vi "SelectRowTablePaste.vi"(7 "エラー入力":errorcluster, 8 "貼り付け指定行":i32, 9 "部分配列":string[][](array[string]), 10 "Tbl refnum":refnum<vi>) -> (0 "エラー出力":errorcluster, 2 "上書データ":string[](array[string]), 3 "リファレンス出力":refnum<vi>)   [LabVIEW 2014]
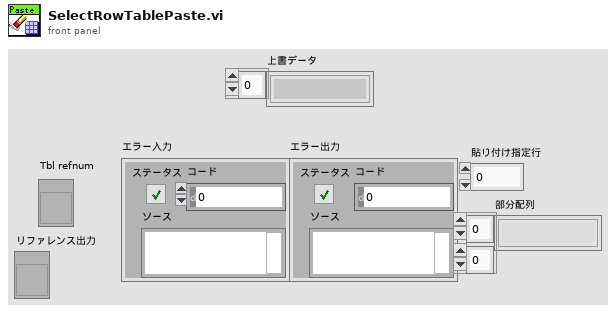
[diagram p1: front panel]
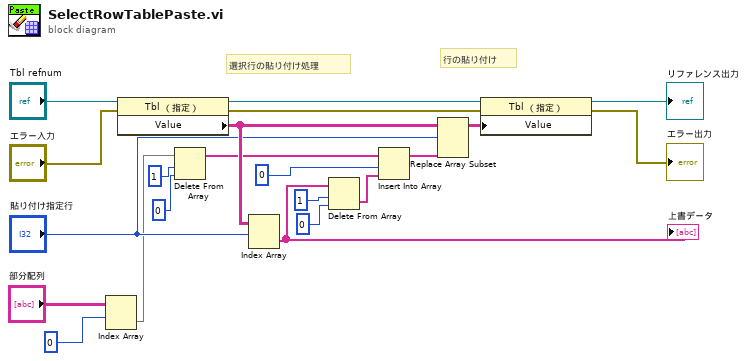
[diagram p0: block diagram]
diagram:
  # "行の貼り付け"
  # "選択行の貼り付け処理"
  n1 = Index Array(array="部分配列", index (row)=0 ("指標 （行）")) -> (element=w10:string[])  [unwired: 1 in]
  n2 = property class="Tbl （指定）"(reference="Tbl refnum", error in="エラー入力") -> (reference out=w17:refnum<vi>, error out=w16:errorcluster, "Value"=w14:string[][])
  n3 = Delete From Array(array=w10, length=1 ("長さ"), index=0 ("指標")) -> (array with subset deleted=w7:string[])  [unwired: 1 out]
  n4 = Index Array(array=w14, index (row)="貼り付け指定行") -> (element=w4:string[])  [unwired: 1 in]
  "上書データ" <- w4
  n5 = Delete From Array(array=w4, length=1 ("長さ"), index=0 ("指標")) -> (deleted portion=w3:string[])  [unwired: 1 out]
  n6 = Insert Into Array(array=w7, index=0 ("指標"), new element=w3) -> (w5:string[])
  n7 = Replace Array Subset(array=w14, new element=w5, index (row)="貼り付け指定行") -> (w15:string[][])  [unwired: 1 in]
  n8 = property class="Tbl （指定）"(reference=w17, error in=w16, "Value"=w15) -> (reference out=→"リファレンス出力":refnum<vi>, error out=→"エラー出力":errorcluster)
